vi "EEPROM_data.vi"() -> (0 "EEPROM Data":T1)   [LabVIEW 2010, in "lib1299.lvlib"]
doc: "This VI serves as a initialized shift register for the data read from the EEPROM programming file."
uses:
  lib1299.lvlib
  Controls/EEPROM_data.ctl
  Controls/EDGE ITEM.ctl
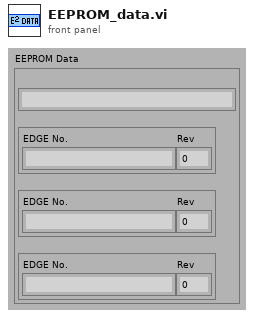
[diagram p1: front panel]
types:
  T1 = typedef "lib1299.lvlib/EEPROM_data.ctl" = cluster{"EVM Name":string, "PWB":T2, "PCA":T2, "BOM":T2}
  T2 = typedef "lib1299.lvlib/EDGE ITEM.ctl" = cluster{"EDGE No.":string, "Rev":u16}
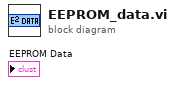
[diagram p0: block diagram]
diagram:
